vi "Transform.vi"(7 "Type X":T1(ring), 8 "error in (no error)":errorcluster caption="entrée d'erreur (pas d'erreur)", 9 "y":string[][](array[string]), 10 "X":string[][](array[string]), 11 "Binarizer en entrée":refnum<class "Binarizer.lvclass">) -> (0 "error out":errorcluster caption="sortie d'erreur", 2 "Data":T2, 3 "Binarizer en sortie":refnum<class "Binarizer.lvclass">)   [LabVIEW 2020, in "Binarizer.lvclass"]
doc: "Binarize each element of X\n\nReturns :\n\n- X_new : ndarray array of shape (n_samples, n_features_new)\nTransformed array."
uses:
  Binarizer.lvclass
  Binarizer.lvclass/Binarizer.ctl
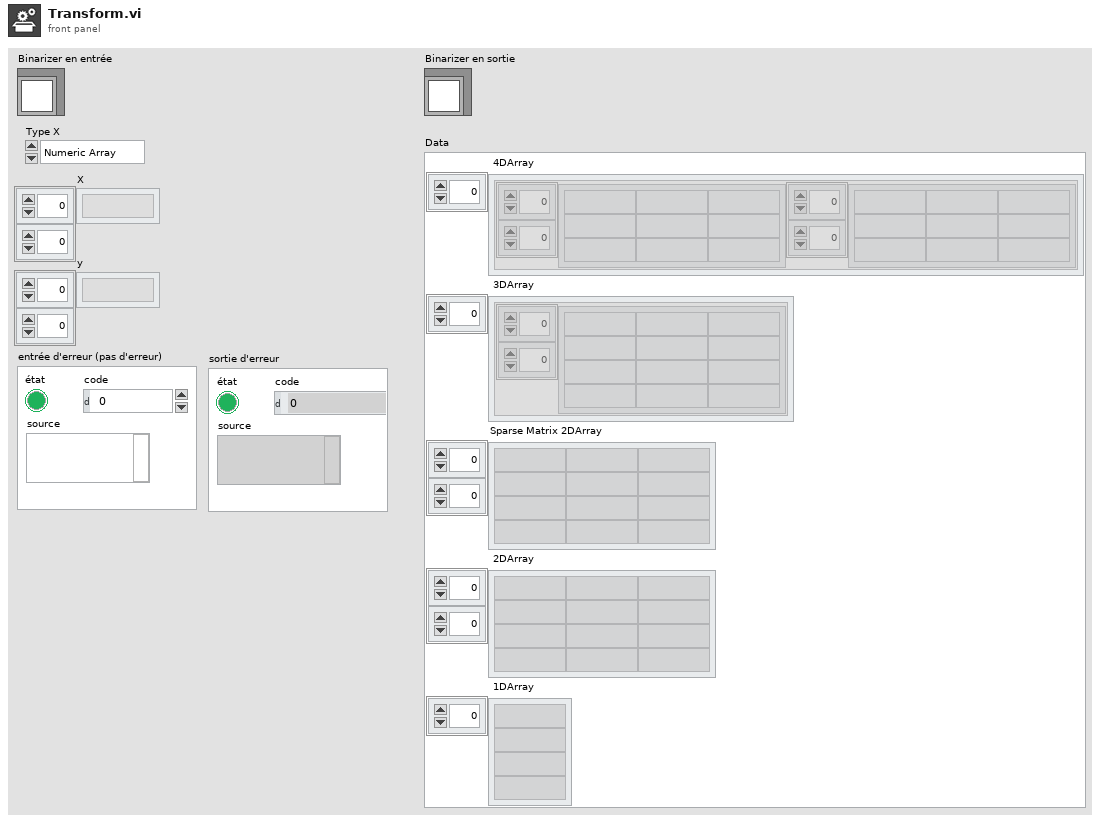
[diagram p1: front panel]
types:
  T1 = enum16{"Numeric Array", "String Array", "Sparse"}
  T2 = cluster{" 4DArray":cluster{"1":string[][], "2":string[][]}[], " 3DArray":cluster{"Tableau":string[][]}[], "Sparse Matrix 2DArray":string[][], " 2DArray":string[][], " 1DArray":string[]}
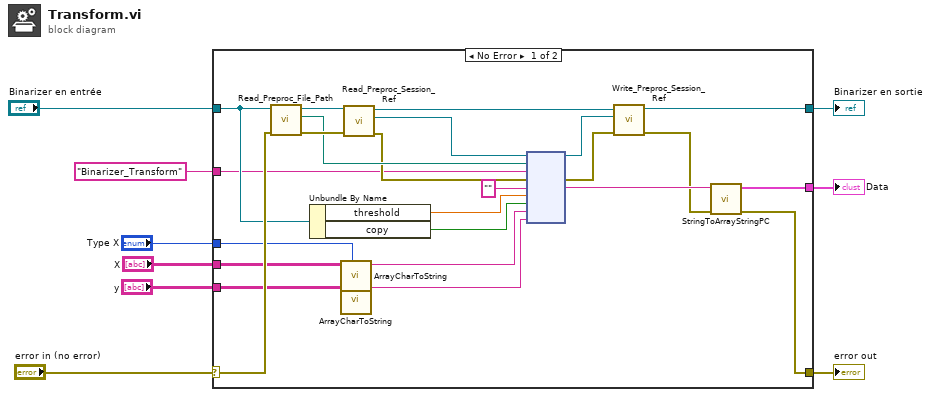
[diagram p0: block diagram]
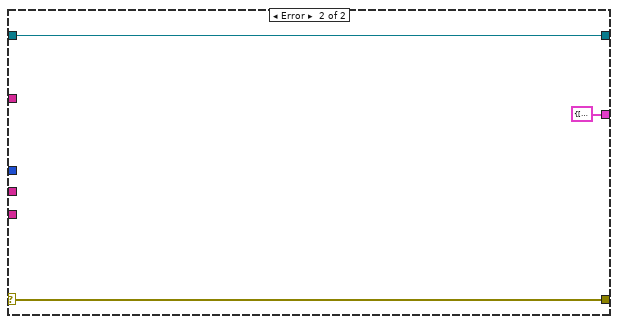
[diagram p2: hidden frame]
diagram:
  n1 = case shown="No Error" "error in (no error)" {
    selector: "error in (no error)" -> [w22 w36]
    tunnel: [w11 w36] -> w8
    tunnel: [w12 w35] -> w6
    tunnel: "Binarizer en entrée" -> [w21 w35]
    tunnel: "X" -> [w19 _]
    tunnel: "y" -> [w18 _]
    tunnel: "Binarizer_Transform" -> [w20 _]
    tunnel: [w13 T2 {" 4DArray"=[], " 3DArray"=[], "Sparse Matrix 2DArray"=[], " 2DArray"=[], " 1DArray"=[]} ("Data")] -> w2
    tunnel: "Type X" -> [w17 _]
    frame No Error {
      n2 = call-dynamic "Read_Preproc_File_Path.vi"("error in (no error)"=w22, "Python in"=w21) -> ("error out"=w32:errorcluster, "File_Path"=w29:path, "Python out"=w33:refnum<class "Binarizer.lvclass">)  [unwired: 7 in]
      n3 = Unbundle By Name(w21) -> ("threshold"=w24:dbl, "copy"=w23:bool)
      n4 = call "ArrayCharToString.vi"("Type"=w17, "TAB"=w19) -> ("Instruction"=w16:string)  [unwired: 9 in]
      n5 = call "ArrayCharToString.vi"("TAB"=w18) -> ("Instruction"=w15:string)  [unwired: 10 in]
      n6 = call-dynamic "Read_Preproc_Session_Ref.vi"("error in (no error)"=w32, "Python in"=w33) -> ("error out"=w28:errorcluster, "Session_ref"=w30:refnum<k35>, "Python out"=w31:refnum<class "Binarizer.lvclass">)  [unwired: 7 in]
      n7 = node(w30, w29, w20, w28, "", w24, w23, w16, w15) -> (w26:refnum<k35>, w27:errorcluster, w14:string)  [unwired: 4 in, 2 out]
      n8 = call-dynamic "Write_Preproc_Session_Ref.vi"("error in (no error)"=w27, "Session_ref"=w26, "Python in"=w31) -> ("error out"=w10:errorcluster, "Python out"=w12:refnum<class "Binarizer.lvclass">)  [unwired: 7 in]
      n9 = call "StringToArrayStringPC.vi"("sortie d'erreur"=w10, "Return value"=w14) -> ("sortie d'erreur"=w11:errorcluster, "Data"=w13:T2)  [unwired: 8 in]
    }
    frame Error {
    }
  }
  "error out" <- w8
  "Binarizer en sortie" <- w6
  "Data" <- w2
